vi "UNO_Detect.vi"(8 "errin":errorcluster) -> (0 "error out":errorcluster, 3 "Visa UNO":refnum<visa-resource-name>)   [LabVIEW 2020]
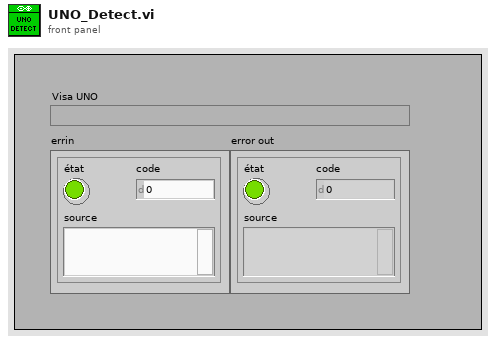
[diagram p1: front panel]
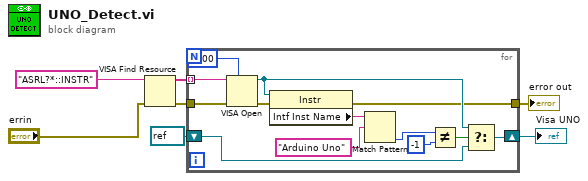
[diagram p0: block diagram]
diagram:
  n1 = VISA Find Resource(8:"errin", 11:"ASRL?*::INSTR" ("expression  (\"?*\")")) -> (0:w4:errorcluster, 3:w5:string[])  [unwired: 1 in, 1 out]
  n2 = for {
    tunnel: w5 -> [w19] mode=indexing
    tunnel: w4 -> [w20]
    shift-right: [w12] -> w2
    shift-left: refnum<visa-resource-name> refnum ("VISA resource name") -> [w11]
    tunnel: [w10] -> w1
    n3 = VISA Open(timeout (0)=u32 1000 ("Timeout de VISA Open (0)"), error in (no error)=w20, VISA resource name=w19) -> (VISA resource name=w13:refnum<visa-resource-name>, error out=w18:errorcluster)  [unwired: 2 in]
    n4 = property class="Instr"(reference=w13, error in=w18) -> (error out=w10:errorcluster, "Intf Inst Name"=w9:string)  [unwired: 1 out]
    n5 = Match Pattern(string=w9, regular expression="Arduino Uno" ("expression régulière")) -> (offset past match=w16:i32)  [unwired: 1 in, 3 out]
    n6 = Not Equal?(x=w16, y=-1) -> (x != y?=w14:bool)
    n7 = Select(t=w13, s=w14, f=w11) -> (s? t:f=w12:refnum<visa-resource-name>)
  }
  "Visa UNO" <- w2
  "error out" <- w1
